vi "subvi_step_motor.vi"(11 "Write to Motor?":cluster{"Analyser 1":bool, "Analyser 2":bool}) -> ()   [LabVIEW 2014]
doc: "This is a program to step a stepper motor with one step of duration 1 millisecond\nCreated on: 15/08/2019\nAuthor: Manish Patel"
panel:
  # "INPUTS"
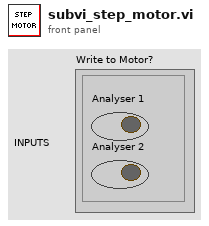
[diagram p1: front panel]
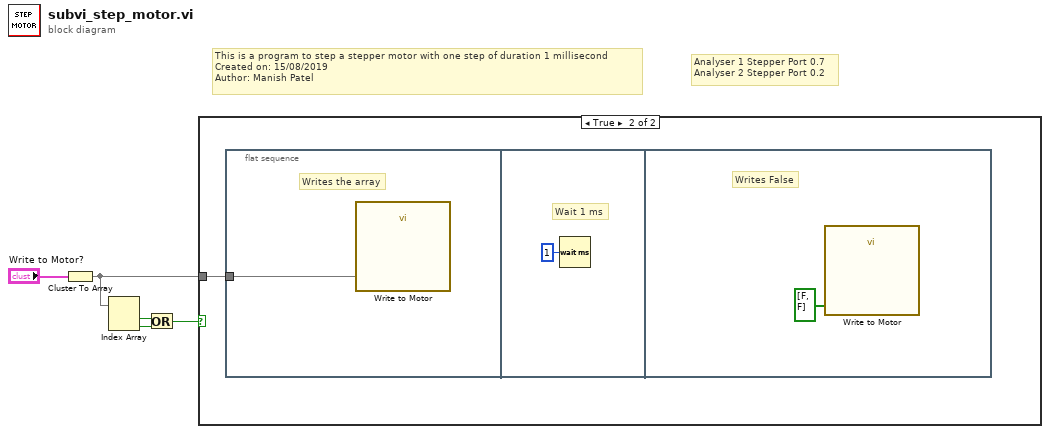
[diagram p0: block diagram]
diagram:
  # "Analyser 1 Stepper Port 0.7\nAnalyser 2 Stepper Port 0.2"
  # "This is a program to step a stepper motor with one step of duration 1 millisecond\nCreated on: 15/08/2019\nAuthor: Manish Patel"
  n1 = Cluster To Array(cluster="Write to Motor?") -> (array=w4:bool[])
  n2 = Index Array(array=w4) -> (element #1=w2:bool, element #2=w3:bool)  [unwired: 2 in]
  n3 = Or(x=w2, y=w3) -> (x .or. y?=w1:bool)
  n4 = case shown="True" w1 {
    tunnel: w4 -> [_ w6]
    frame False {
    }
    frame True {
      n5 = flat-sequence {
        tunnel: w6 -> [w7]
        frame #0 {
          # "Writes the array"
          n6 = call "Write to Motor"("data"=w7) -> ()  [unwired: 17 in, 2 out]
        }
        frame #1 {
          # "Wait 1 ms"
          n7 = Wait (ms)(milliseconds to wait=u32 1) -> ()  [unwired: 1 out]
        }
        frame #2 {
          # "Writes False"
          n8 = call "Write to Motor"("data"=bool[] [FALSE, FALSE]) -> ()  [unwired: 17 in, 2 out]
        }
      }
    }
  }
